vi "Initialize.vi"(4 "FIFO Options":T1, 5 "Status":refnum<class "Framework Status.lvclass">, 6 "id":i32, 7 "Logging Interface":refnum<class "Logging Interface.lvclass">, 8 "error in (no error)":errorcluster, 9 "Transfer Groups":refnum<class "Transfer Group.lvclass">[](array[class]), 10 "Components":refnum<class "Component.lvclass">[](array[class]), 11 "Plugin Configuration":refnum<class "Plugin Configuration.lvclass">) -> (0 "error out":errorcluster, 2 "Plugin Threads":refnum<class "Plugin Thread.lvclass">[](array[class]), 3 "Plugin out":refnum<class "Plugin.lvclass">)   [LabVIEW 2020, in "DSF Core.lvlib" / "Plugin.lvclass"]
uses:
  Plugin.lvclass
  Timing/Timing.lvclass
  Configuration/Core/Plugin/Plugin Configuration.lvclass
  Framework Status/Framework Status.lvclass
  Thread/Plugin/Plugin Thread.lvclass
  Typedefs/DSF FIFO Options.ctl
  Framework/Framework.lvclass
  Interface/Logging/Logging Interface.lvclass
  Component/Component.lvclass
  Transfer Group/Transfer Group.lvclass
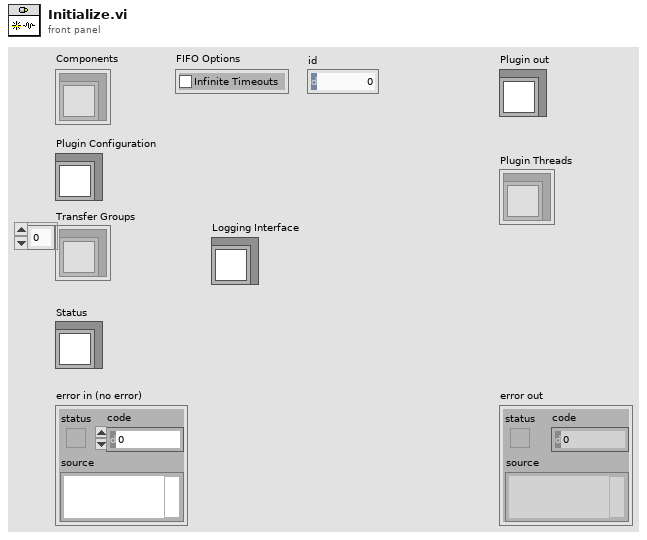
[diagram p1: front panel]
types:
  T1 = typedef "DSF Core.lvlib/Framework.lvclass/DSF FIFO Options.ctl" = cluster{"Infinite Timeouts":bool}
  T2 = typedef "DSF Core.lvlib/Plugin Configuration.lvclass/Core Plugin Configuration.ctl" = cluster{"name":string, "components":string[], "cycle timing":T3}
  T3 = typedef "DSF Core.lvlib/DSF Timing Info.ctl" = cluster{"priority":u64, "decimation":u64, "offset":u64}
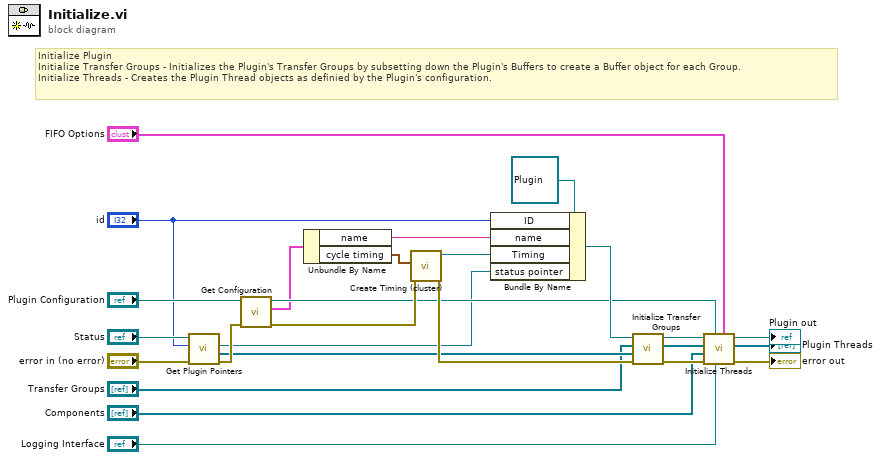
[diagram p0: block diagram]
diagram:
  # "Initialize Plugin\nInitialize Transfer Groups - Initializes the Plugin's Transfer Groups by subsetting down the Plugin's Buffers to create a Buffer object for each Group.\nInitialize Threads - Creates the Plugin Thread objects as definied by the Plugin's configuration."
  n1 = call "Get Plugin Pointers.vi"("error in (no error)"="error in (no error)", "plugin index"="id", "Framework Status in"="Status") -> ("error out"=w8:errorcluster, "group status pointers"=w4:refnum<class "Status Pointer.lvclass">[], "plugin status pointer"=w5:refnum<class "Status Pointer.lvclass">)  [unwired: 5 in, 1 out]
  n2 = call "Get Configuration.vi"("error in (no error)"=w8, "Core Plugins Configuration in"="Plugin Configuration") -> ("error out"=w7:errorcluster, "configuration"=w2:T2, "Core Plugins Configuration out"=w6:refnum<class "Plugin Configuration.lvclass">)  [unwired: 7 in]
  n3 = Unbundle By Name(w2) -> ("name"=w14:string, "cycle timing"=w13:T3)
  n4 = call "Create Timing (cluster).vi"("error in (no error)"=w7, "cycle timing"=w13) -> ("error out"=w17:errorcluster, "Timing"=w20:refnum<class "Timing.lvclass">)  [unwired: 8 in]
  n5 = Bundle By Name(cluster=refnum<class "Plugin.lvclass"> refnum ("DSF Core.lvlib:Plugin"), "ID"="id", "name"=w14, "Timing"=w20, "status pointer"=w5) -> (w19:refnum<class "Plugin.lvclass">)
  n6 = call "Initialize Transfer Groups.vi"("error in (no error)"=w17, "group status pointers"=w4, "Transfer Groups in"="Transfer Groups", "Plugin in"=w19) -> ("error out"=w23:errorcluster, "Transfer Groups out"=w15:refnum<class "Transfer Group.lvclass">[], "Plugin out"=w25:refnum<class "Plugin.lvclass">)  [unwired: 5 in]
  n7 = call "Initialize Threads.vi"("FIFO Options"="FIFO Options", "Logging Interface"="Logging Interface", "Plugin Configuration"=w6, "error in (no error)"=w23, "Components"="Components", "Transfer Groups"=w15, "Plugin in"=w25) -> ("error out"=→"error out":errorcluster, "Plugin Threads"=→"Plugin Threads":refnum<class "Plugin Thread.lvclass">[], "Plugin out"=→"Plugin out":refnum<class "Plugin.lvclass">)  [unwired: 2 in]
